vi "TR_ManageContextMenu.vi"(8 "error in (no error)":errorcluster, 11 "Menu in":refnum<class "Menu.lvclass">) -> (0 "error out":errorcluster)   [LabVIEW 2021, in "Menu.lvlib" / "Menu.lvclass"]
uses:
  Menu.lvclass
  Menu.lvclass/Menu.ctl
  <vilib>/event_ctls.llb/usereventprio.ctl
  InputDevice/src/Mouse/Mouse.lvclass
  InputDevice/src/Keyboard/Keyboard.lvclass
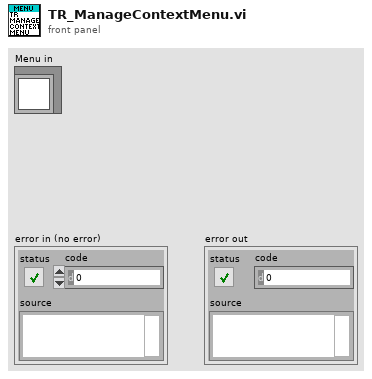
[diagram p1: front panel]
types:
  T1 = cluster{"Mouse":refnum<event-registration>, "Keyboard":refnum<event-registration>, "Event Registration Refnum":refnum<event-registration>}
  T2 = typedef "usereventprio.ctl" = enum32{"high priority", "normal priority"}
  T3 = typedef "LVPoint32TypeDef.ctl" = cluster{"Horizontal":i32, "Vertical":i32}
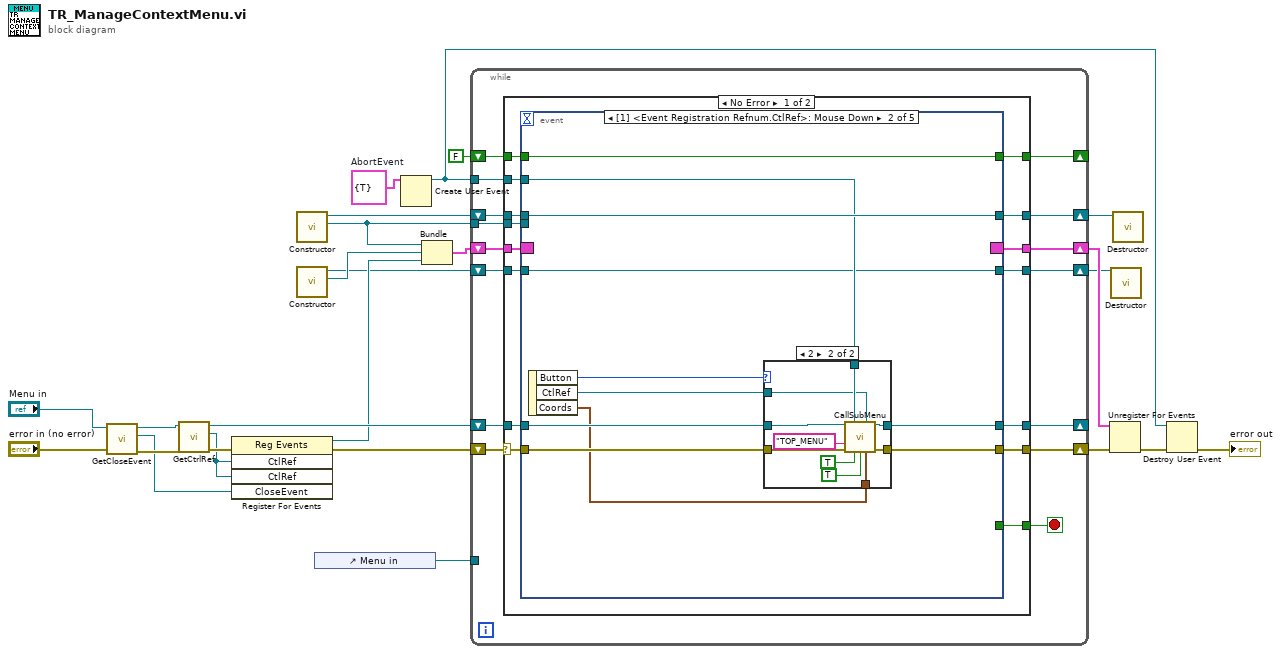
[diagram p0: block diagram]
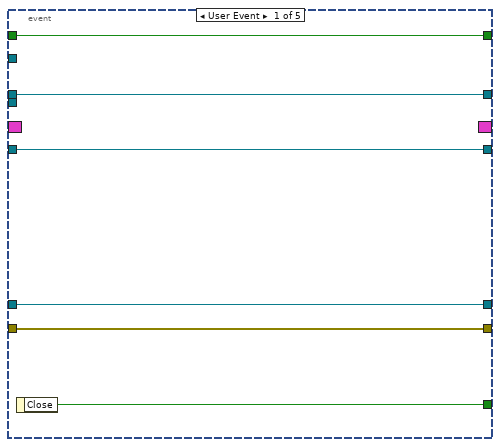
[diagram p2: hidden frame]
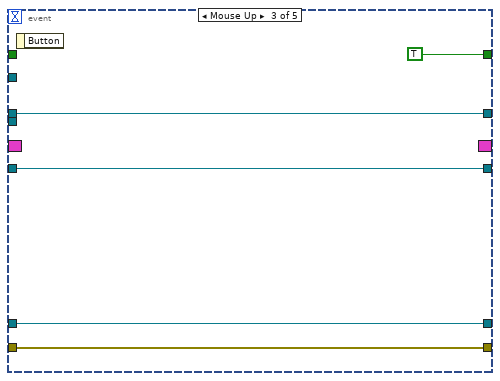
[diagram p4: hidden frame]
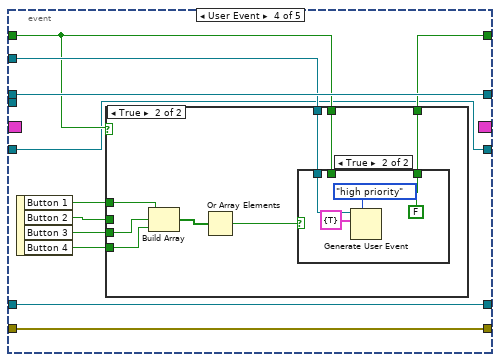
[diagram p5: hidden frame]
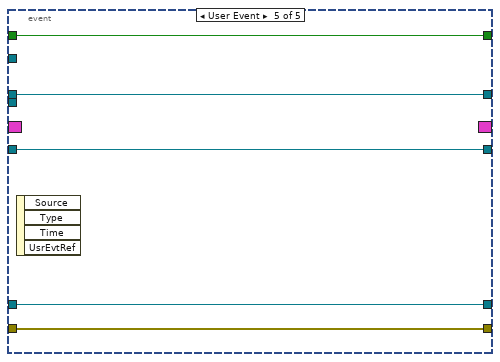
[diagram p8: hidden frame]
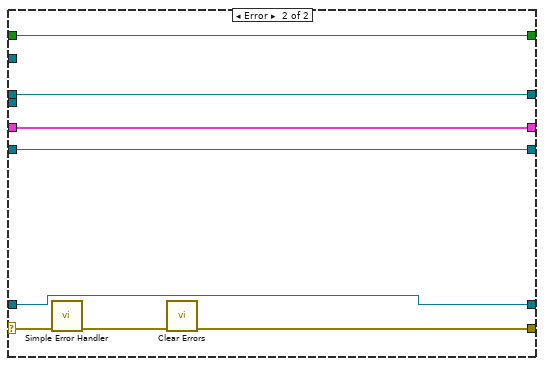
[diagram p9: hidden frame]
diagram:
  w20 = cluster{"Abort":bool} {"Abort"=TRUE}  # AbortEvent
  n1 = call "GetCloseEvent.vi"("error in (no error)"="error in (no error)", "Menu in"="Menu in") -> ("error out"=w11:errorcluster, "CloseEvent"=w5:refnum<user-event>, "Menu out"=w13:refnum<class "Menu.lvclass">)  [unwired: 7 in]
  n2 = call "GetCtrlRef.vi"("error in (no error)"=w11, "Menu in"=w13) -> ("error out"=w10:errorcluster, "CtlRef"=w6:refnum<vi>, "Menu out"=w9:refnum<class "Menu.lvclass">)  [unwired: 7 in]
  n3 = register-events(error in=w10, w6, w6, w5) -> (reference out=w3:refnum<event-registration>, error out=w8:errorcluster)  [unwired: 1 in]
  n4 = call "Constructor.vi"() -> ("Mouse"=w15:refnum<event-registration>, "Mouse out"=w22:refnum<class "Mouse.lvclass">)  [unwired: 9 in, 1 out]
  n5 = call "Constructor.vi"() -> ("Keyboard"=w4:refnum<event-registration>, "Keyboard out"=w2:refnum<class "Keyboard.lvclass">)  [unwired: 9 in, 1 out]
  n6 = control-ref of="Menu in"() -> (w16:refnum<vi>)
  n7 = Create User Event(user event datatype=w20) -> (user event=w25:refnum<user-event>)  [unwired: 1 in, 1 out]
  n8 = Bundle("Mouse"=w15, "Keyboard"=w4, "Event Registration Refnum"=w3) -> (w21:T1)  [unwired: 1 in]
  n9 = while {
    shift-right: [w37] -> _
    shift-left: w9 -> [w40]
    tunnel: w25 -> [w34]
    shift-right: [w32] -> _
    shift-left: FALSE -> [w33]
    shift-right: [w30] -> w23
    shift-left: w22 -> [w31]
    shift-right: [w35] -> w19
    shift-left: w21 -> [w36]
    shift-right: [w38] -> w17
    shift-left: w8 -> [w39]
    tunnel: w16 -> [_]
    tunnel: w15 -> [w28]
    shift-right: [w26] -> w1
    shift-left: w2 -> [w27]
    stop <- w29 stop-if-true
    n10 = case shown="No Error" w39 {
      selector: w39 -> [w54 w127]
      tunnel: w40 -> [w55 w126]
      tunnel: [w53 w124] -> w38
      tunnel: [w52 w126] -> w37
      tunnel: w36 -> [w51 w123]
      tunnel: [w50 w123] -> w35
      tunnel: w34 -> [w49 _]
      tunnel: w33 -> [w48 w122]
      tunnel: [w47 w122] -> w32
      tunnel: w31 -> [w46 w121]
      tunnel: [w45 w121] -> w30
      tunnel: [w44 _] -> w29
      tunnel: w28 -> [w43 _]
      tunnel: w27 -> [w42 w120]
      tunnel: [w41 w120] -> w26
      frame No Error {
        n11 = event shown="[1] <Event Registration Refnum.CtlRef>: Mouse Down" {
          selector: w51 -> [_ _ _ _ _]
          dyn-events: [_ _ _ _ _] -> w50
          timeout: _ -> [_ _ _ _ _]
          tunnel: w55 -> [w61 w68 w88 w100 w118]
          tunnel: w54 -> [w58 w67 w89 w93 w119]
          tunnel: [w58 w72 w89 w93 w119] -> w53
          tunnel: [w61 w71 w88 w100 w118] -> w52
          tunnel: w49 -> [_ w69 _ w94 _]
          tunnel: w48 -> [w60 w65 _ w91 w117]
          tunnel: [w60 w65 TRUE w92 w117] -> w47
          tunnel: w46 -> [w59 w70 w87 w99 w116]
          tunnel: [w59 w70 w87 w99 w116] -> w45
          tunnel: [w57 _ _ _ _] -> w44
          tunnel: w43 -> [_ _ _ _ _]
          tunnel: w42 -> [w56 w62 w85 w90 w115]
          tunnel: [w56 w62 w85 w90 w115] -> w41
          event User Event {
            n12 = event-data() -> ("Close"=w57:bool)  [unwired: 1 in]
          }
          event Mouse Down {
            n13 = event-data() -> ("Button"=w64:u16, "CtlRef"=w66:refnum<vi>, "Coords"=w63:T3)  [unwired: 1 in]
            n14 = case shown="2" w64 {
              tunnel: [w73 w84] -> w72
              tunnel: [w74 w83] -> w71
              tunnel: w69 -> [_ w82]
              tunnel: w68 -> [w74 w81]
              tunnel: w67 -> [w73 w80]
              tunnel: w66 -> [_ w79]
              tunnel: w63 -> [_ w77]
              frame 0, Default {
              }
              frame 2 {
                n15 = call "CallSubMenu.vi"("Menu in"=w81, "User Event"=w82, "CtrlRef"=w79, "Selected Tag"="TOP_MENU", "error in (no error)"=w80, "SubMenu"=TRUE, "ContextMenu"=TRUE, "Coords"=w77) -> ("Menu out"=w83:refnum<class "Menu.lvclass">, "error out"=w84:errorcluster)  [unwired: 6 in]
              }
            }
          }
          event Mouse Up {
            n16 = event-data() -> ()  [unwired: 1 in, 1 out]
          }
          event User Event {
            n17 = event-data() -> ("Button 1"=w98:bool, "Button 2"=w97:bool, "Button 3"=w96:bool, "Button 4"=w95:bool)  [unwired: 1 in]
            n18 = case shown="True" w91 {
              tunnel: w98 -> [_ w109]
              tunnel: w97 -> [_ _]
              tunnel: w96 -> [_ w102]
              tunnel: w95 -> [_ w108]
              tunnel: w94 -> [_ w106]
              tunnel: [w101 w104] -> w92
              tunnel: w91 -> [w101 w103]
              frame False {
              }
              frame True {
                n19 = Build Array(w109, w102, w108) -> (w107:bool[])
                n20 = Or Array Elements(Boolean array=w107) -> (logical OR=w105:bool)
                n21 = case shown="True" w105 {
                  tunnel: w106 -> [_ w114]
                  tunnel: [w110 FALSE] -> w104
                  tunnel: w103 -> [w110 _]
                  frame False {
                  }
                  frame True {
                    n22 = Generate User Event(priority (normal)=usereventprio."high priority", user event=w114, event data cluster=cluster{"Abort":bool} {"Abort"=TRUE} ("event data")) -> ()  [unwired: 1 in, 2 out]
                  }
                }
              }
            }
          }
          event User Event {
            n23 = event-data() -> ()  [unwired: 1 in, 4 out]
          }
        }
      }
      frame Error {
        n24 = call <vilib>:"Simple Error Handler.vi"("error in (no error)"=w127) -> ("error out"=w125:errorcluster)  [unwired: 4 in, 4 out]
        n25 = call <vilib>:"Clear Errors.vi"("error in (no error)"=w125) -> ("error out"=w124:errorcluster)  [unwired: 5 in, 1 out]
      }
    }
  }
  n26 = Unregister For Events(event registration refnum=w19, error in=w17) -> (error out=w18:errorcluster)
  n27 = call-dynamic "Destructor.vi"("Mouse in"=w1) -> ()  [unwired: 10 in, 1 out]
  n28 = call-dynamic "Destructor.vi"("Mouse in"=w23) -> ()  [unwired: 10 in, 1 out]
  n29 = Destroy User Event(user event=w25, error in=w18) -> (error out=→"error out":errorcluster)
